vi "Record_Front_Panel.vi"(1 "VI to Log":path) -> ()   [LabVIEW 2020]
uses:
  Globals/Meas_global.vi
panel:
  in  "Folder to log to":path
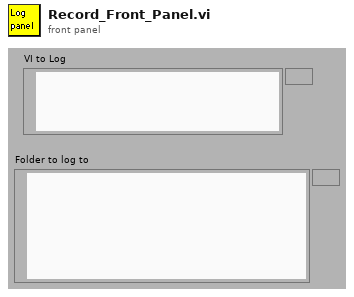
[diagram p1: front panel]
types:
  T1 = enum32{"existing file", "new file", "new or existing file", "existing dir", "new dir", "new or existing dir", "existing file (use LLBs)", "new file (use LLBs)", "new or existing file (use LLBs)", "new or existing file or directory (use LLBs)"}
  T2 = typedef "LVRectTypeDef.ctl" = cluster{"left":i16, "top":i16, "right":i16, "bottom":i16}
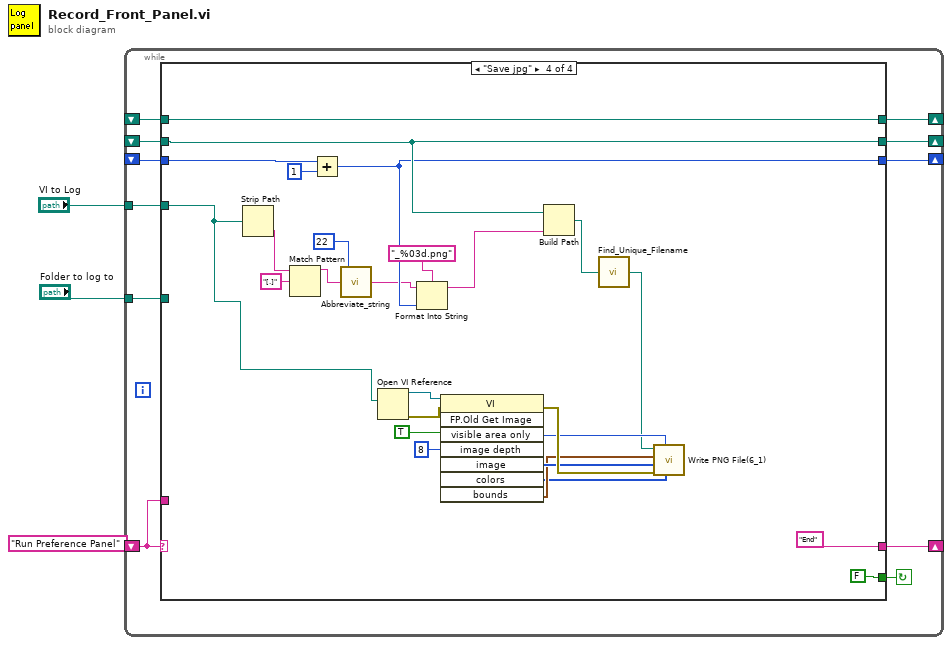
[diagram p0: block diagram]
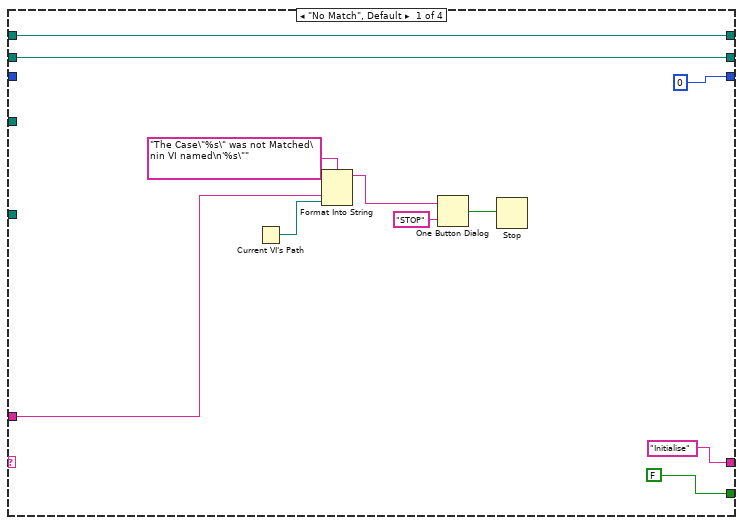
[diagram p2: hidden frame]
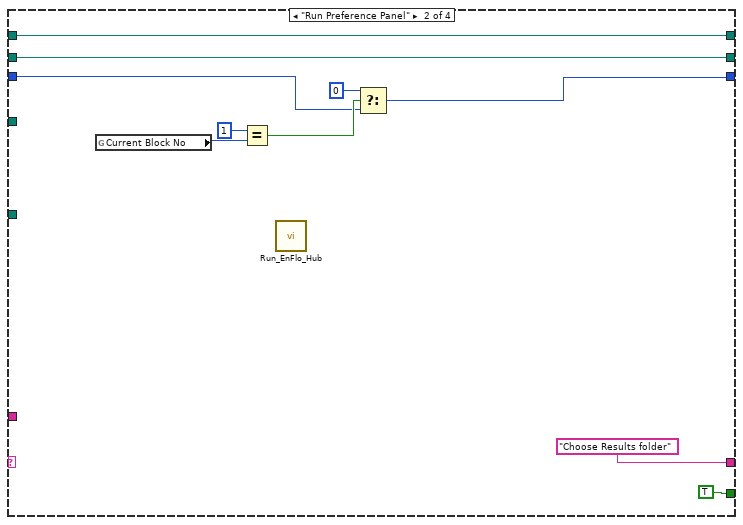
[diagram p3: hidden frame]
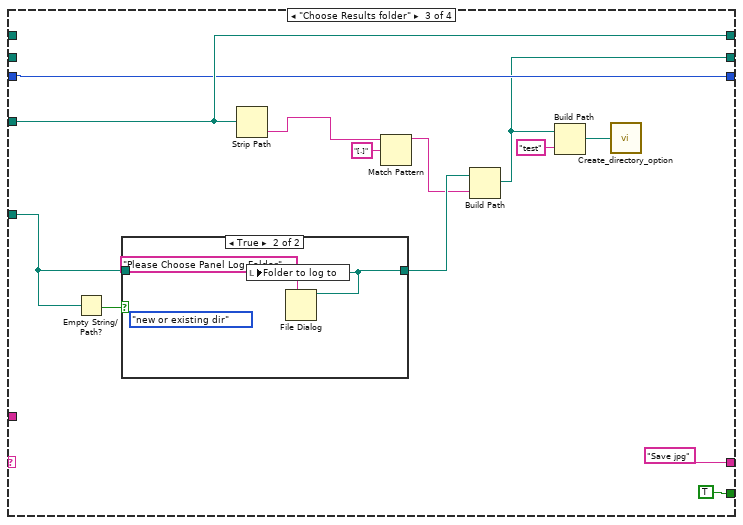
[diagram p4: hidden frame]
diagram:
  n1 = while {
    shift-left: "Run Preference Panel" -> [w12]
    shift-right: [w13] -> _
    shift-right: [w8] -> _
    shift-left: _ -> [w9]
    tunnel: "Folder to log to" -> [w11]
    tunnel: "VI to Log" -> [w10]
    shift-right: [w7] -> _
    shift-left: _ -> [w6]
    shift-right: [w5] -> _
    shift-left: _ -> [w4]
    stop <- w14 continue-if-true
    n2 = case shown="\"Save jpg\"" w12 {
      tunnel: [FALSE TRUE TRUE FALSE] -> w14
      tunnel: ["Initialise" "Choose Results folder" "Save jpg" "End"] -> w13
      tunnel: w12 -> [w20 _ _ _]
      tunnel: w11 -> [_ _ w45 _]
      tunnel: w10 -> [_ _ w43 w57]
      tunnel: w9 -> [w17 w34 _ w74]
      tunnel: [w17 w34 w43 w74] -> w8
      tunnel: [w16 w33 w41 w72] -> w7
      tunnel: w6 -> [w16 w33 _ w72]
      tunnel: [0 w27 w42 w69] -> w5
      tunnel: w4 -> [_ w28 w42 w71]
      frame "No Match", Default {
        n3 = Current VI's Path() -> (path=w19:path)
        n4 = Format Into String(format string="The Case\"%s\" was not Matched\nin VI named\n'%s\"" ("Format String"), w20, w19) -> (resulting string=w23:string)  [unwired: 2 in, 1 out]
        n5 = One Button Dialog(message=w23, button name ("OK")="STOP") -> (true=w21:bool)
        n6 = Stop(stop? (T)=w21) -> ()
      }
      frame "Run Preference Panel" {
        n7 = global read "Meas_global.vi" "Current Block No"() -> (w31:i32)
        n8 = Equal?(x=1, y=w31) -> (x = y?=w29:bool)
        n9 = call "Run_EnFlo_Hub.vi"() -> ()  [unwired: 1 in, 7 out]
        n10 = Select(t=0, s=w29, f=w28) -> (s? t:f=w27:i32)
      }
      frame "Choose Results folder" {
        n11 = Empty String/Path?(string/path=w45) -> (empty?=w46:bool)
        n12 = case shown="True" w46 {
          tunnel: [w49 w51] -> w44
          tunnel: w45 -> [w49 _]
          frame False {
          }
          frame True {
            (unwired) T1."new or existing dir" ("select mode (2)")
            n13 = File Dialog(7:"Please Choose Panel Log Folder" ("prompt")) -> (3:w51:path)  [unwired: 1 in, 8 out]
            n14 = local write "Folder to log to"(w51) -> ()
          }
        }
        n15 = Strip Path(path=w43) -> (name=w37:string)  [unwired: 1 out]
        n16 = Match Pattern(string=w37, regular expression="[.]") -> (before substring=w36:string)  [unwired: 4 out]
        n17 = Build Path(base path=w44, name or relative path=w36) -> (appended path=w41:path)
        n18 = Build Path(base path=w41, name or relative path="test") -> (appended path=w39:path)
        n19 = call "Create_directory_option.vi"("Filename"=w39) -> ()  [unwired: 2 out]
      }
      frame "Save jpg" {
        w58 = 8 ("image depth")
        n20 = Strip Path(path=w57) -> (name=w67:string)  [unwired: 1 out]
        n21 = Match Pattern(string=w67, regular expression="[.]") -> (before substring=w56:string)  [unwired: 4 out]
        n22 = Add(x=w71, y=1) -> (x+y=w69:i32)
        n23 = call "Abbreviate_string.vi"("Input String"=w56, "Max String Length"=22) -> ("Output String"=w54:string)  [unwired: 1 in, 2 out]
        n24 = Open VI Reference(vi path=w57) -> (vi reference=w65:refnum<vi>, error out=w64:errorcluster)  [unwired: 1 in, 4 out]
        n25 = Format Into String(format string="_%03d.png", initial string=w54, w69) -> (resulting string=w73:string)  [unwired: 1 in, 1 out]
        n26 = invoke class="VI" method="FP.Old Get Image"(reference=w65, error in=w64, "visible area only"=TRUE, "image depth"=w58) -> (error out=w62:errorcluster, "image"=w61:u8[], "colors"=w59:u32[], "bounds"=w60:T2)  [unwired: 4 in, 4 out]
        n27 = Build Path(base path=w72, name or relative path=w73) -> (appended path=w53:path)
        n28 = call "Find_Unique_Filename.vi"("Path In"=w53) -> ("Unique Path Out"=w52:path)  [unwired: 2 in]
        n29 = call <vilib>:"Write PNG File(6_1).vi"("color table"=w59, "depth"=w58, "error in (no error)"=w62, "flattened image data"=w61, "rect"=w60, "path to PNG file"=w52) -> ()  [unwired: 6 out]
      }
    }
  }
